vi "PH_ImageStatistician.ProcEvents.vi"(0 "i ref in":refnum<vi>, 5 "error in (no error)":errorcluster) -> (14 "i ref out":refnum<vi>, 19 "error out":errorcluster)   [LabVIEW 2014, in "PH_ImageStatistician.lvlib"]
doc: "This method is used to define the events the object will listen to. Add your own events here."
uses:
  PH_ImageStatistician.lvlib
  CS_Core/BaseProcess/BaseProcess.event definition.ctl
  CS_Core/CAEObj/CAEObj.event definition.ctl
  CS_Core/BaseProcess/BaseProcess.descriptor string definition.ctl
  CS_Core/BaseProcess/BaseProcess.lvlib
  CS_Core/CAEObj/CAEObj.lvlib
  PH_Basics/PH_Common/PH_Common.lvlib
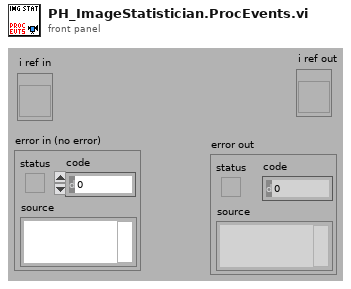
[diagram p1: front panel]
types:
  T1 = typedef "BaseProcess.lvlib/BaseProcess.event definition.ctl" = cluster{"CAEEvtDef":T2, "Data Descriptor":T3}
  T2 = typedef "CAEObj.lvlib/CAEObj.event definition.ctl" = cluster{"URL":string, "enable":bool, "ignoreResID":bool}
  T3 = typedef "BaseProcess.lvlib/BaseProcess.descriptor string definition.ctl" = string
  T4 = typedef "PH_ImageStatistician.lvlib/PH_ImageStatistician.i attribute.ctl" = cluster{"GUI Refs ":cluster{"Status":refnum<vi>, "Result Graph":refnum<vi>, "Mean Data 1":refnum<vi>, "Std Dev Data 1":refnum<vi>, "Mean Data 2":refnum<vi>, "Std Dev Data 2":refnum<vi>, "Mean Data 3":refnum<vi>, "Std Dev Data 3":refnum<vi>, "Dummy Mean":refnum<vi>, "Dummy Std Dev":refnum<vi>, "Export Data":refnum<vi>, "Data 1":refnum<vi>, "Data 2":refnum<vi>, "Data 3":refnum<vi>, "Stat or Trend":refnum<vi>, "Delete":refnum<vi>, "Operator":refnum<vi>, "Start":refnum<vi>}, "Operator":string, "Data":T5[], "Stat or Trend":bool, "Data 1":T6, "Data 2":T6, "Data 3":T6, "Start":bool, "Datasets strored":i32, "Dataarray Size":i32}
  T5 = typedef "PH_ImageStatistician.lvlib/PH_ImageStatistician.Statistician Data.ctl" = cluster{"Snapshot Time":dbl, "Maj FWHM":dbl, "Min FWHM":dbl, "Maj Fit Order":dbl, "Min Fit Order":dbl, "99% Diam Maj Trace":dbl, "99% Diam Min Trace":dbl, "Theta":dbl, "Delta":dbl, "Maj Diam":dbl, "Min Diam":dbl, "Azimuth Angle":dbl, "Azi Angle rel to major?":dbl, "Ellipticity":dbl, "CoG - X":dbl, "CoG - Y":dbl, "Energy":dbl, "Energy Cal - no mJ":dbl, "Lin Cal - no mm or mrad":dbl, "Lin Cal Factor":dbl}
  T6 = typedef "PH_ImageStatistician.lvlib/PH_ImageStatistician.select Data.ctl" = u16
  T7 = typedef "PH_Common.lvlib/PH_DIM.Event Declarer.ctl" = cluster{"Service Name":string, "Selector":string}
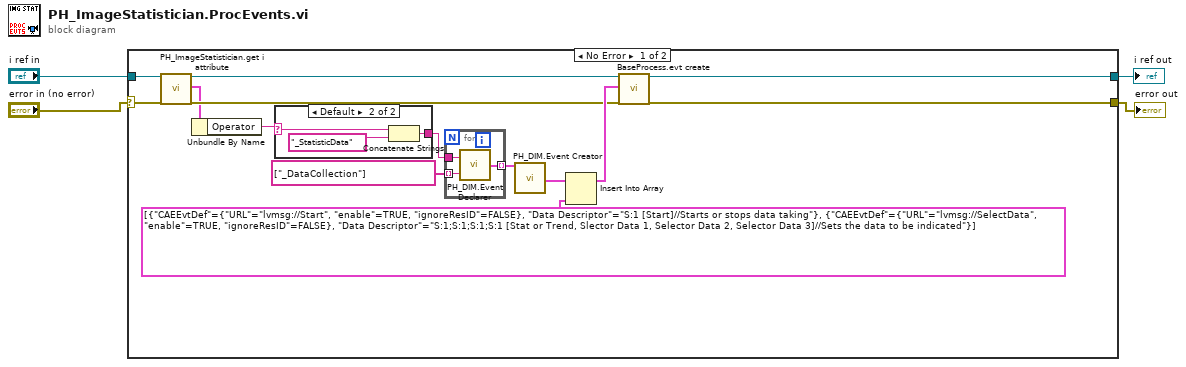
[diagram p0: block diagram]
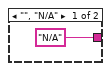
[diagram p2: hidden frame]
diagram:
  n1 = case shown="No Error" "error in (no error)" {
    selector: "error in (no error)" -> [w13 w27]
    tunnel: "i ref in" -> [w11 w26]
    tunnel: [w18 w26] -> w3
    tunnel: [w17 w27] -> w2
    frame No Error {
      n2 = call "PH_ImageStatistician.get i attribute.vi"("i ref in"=w11, "error in (no error)"=w13) -> ("i ref out"=w10:refnum<vi>, "i attribute"=w8:T4, "error out"=w12:errorcluster)  [unwired: 15 in]
      n3 = Unbundle By Name(w8) -> ("Operator"=w7:string)
      n4 = case shown="Default" w7 {
        selector: w7 -> [_ w22]
        tunnel: ["N/A" w21] -> w6
        frame "", "N/A" {
        }
        frame Default {
          n5 = Concatenate Strings(w22, "_StatisticData") -> (w21:string)
        }
      }
      n6 = for {
        tunnel: [w25] -> w5 mode=indexing
        tunnel: w6 -> [w24]
        tunnel: string[] ["_DataCollection"] -> [w23] mode=indexing
        n7 = call "PH_DIM.Event Declarer.vi"("Selector"=w23, "Service Name"=w24) -> ("declared DIM Event"=w25:T7)
      }
      n8 = call "PH_DIM.Event Creator.vi"("Trendnotifier Services"=w5) -> ("DIM Service Events"=w16:T1[])  [unwired: 18 in]
      n9 = Insert Into Array(array=w16, new element=T1[] [{"CAEEvtDef"={"URL"="lvmsg://Start", "enable"=TRUE, "ignoreResID"=FALSE}, "Data Descriptor"="S:1 [Start]//Starts or stops data taking"}, {"CAEEvtDef"={"URL"="lvmsg://SelectData", "enable"=TRUE, "ignoreResID"=FALSE}, "Data Descriptor"="S:1;S:1;S:1;S:1 [Stat or Trend, Slector Data 1, Selector Data 2, Selector Data 3]//Sets the data to be indicated"}] ("new events")) -> (w15:T1[])  [unwired: 1 in]
      n10 = call "BaseProcess.evt create.vi"("i ref in"=w10, "newEvents"=w15, "error in (no error)"=w12) -> ("i ref out"=w18:refnum<vi>, "error out"=w17:errorcluster)  [unwired: 13 in, 2 out]
    }
    frame Error {
    }
  }
  "i ref out" <- w3
  "error out" <- w2
